vi "CheckCom2.vi"(11 "Data In":T2) -> (2 "States":T1, 3 "Data Out":T2)   [LabVIEW 2014]
uses:
  controls/Data.ctl
  controls/State.ctl
panel:
  # "日期"
  # "機種名稱"
  # "機種代號"
  # "商品條碼"
  # "台"
  # "OK"
  # "NG"
  # "台"
  # "總計"
  # "台"
  # "日期"
  # "機種名稱"
  # "機種代號"
  # "商品條碼"
  # "台"
  # "OK"
  # "NG"
  # "台"
  # "總計"
  # "台"
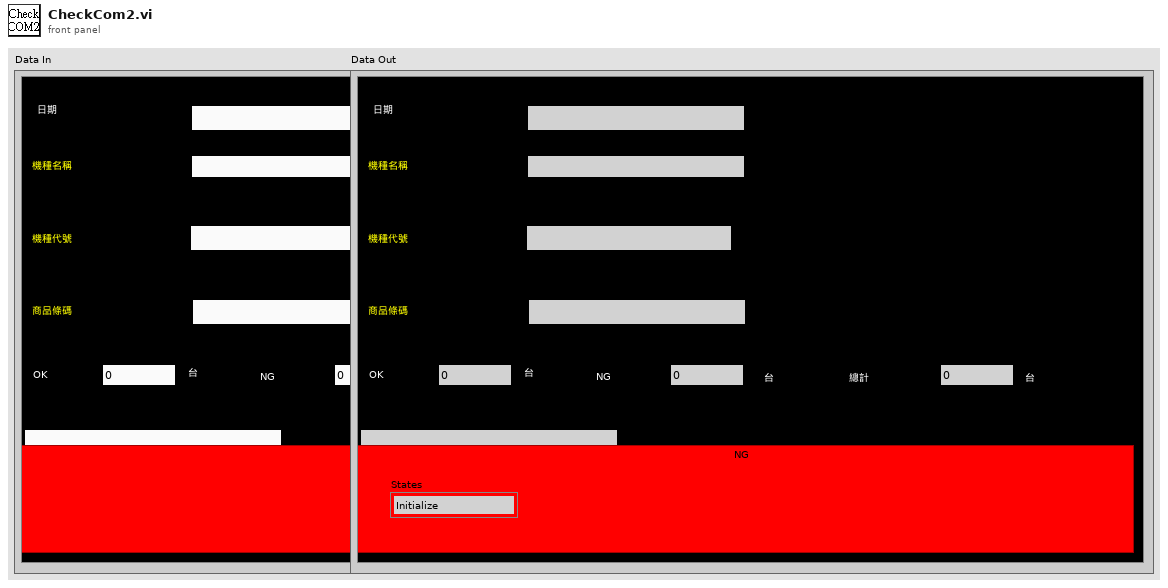
[diagram p1: front panel]
types:
  T1 = typedef "State.ctl" = enum16{"Initialize", "Wait for Scan", "State 1", "State 2", "NG", "OK", "OKNG", "Exit"}
  T2 = typedef "Data.ctl" = cluster{"Date":string, "BarCode1":string, "BarCode2":string, "BarCode3":string, "Message":string, "OK Count":u16, "NG Count":u16, "Total Count":u16, "ModelData":string[][], "OK&NG":bool, "COM1":refnum<visa-resource-name>, "COM2":refnum<visa-resource-name>, "IO":i32, "Time":u32, "TCP":refnum<k5>, "TCP 2":refnum<k5>}
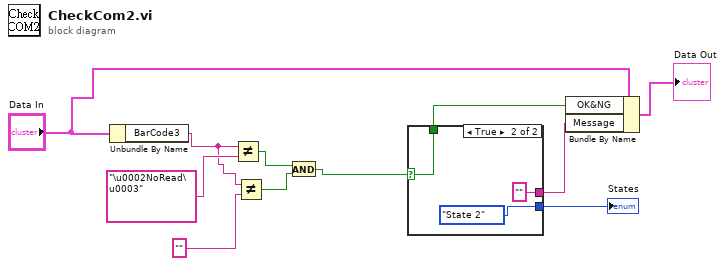
[diagram p0: block diagram]
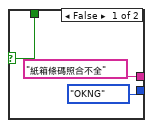
[diagram p2: hidden frame]
diagram:
  n1 = Unbundle By Name("Data In") -> ("BarCode3"=w5:string)
  n2 = Not Equal?(x=w5, y="\u0002NoRead\u0003") -> (x != y?=w3:bool)
  n3 = Not Equal?(x=w5, y="" ("f")) -> (x != y?=w2:bool)
  n4 = And(x=w3, y=w2) -> (x .and. y?=w1:bool)
  n5 = case shown="True" w1 {
    selector: w1 -> [w14 w17]
    tunnel: [w14 w17] -> w9
    tunnel: ["紙箱條碼照合不全" ""] -> w8
    tunnel: [State."OKNG" ("States") State."State 2" ("States")] -> w7
    frame False {
    }
    frame True {
    }
  }
  "States" <- w7
  n6 = Bundle By Name(cluster="Data In", "OK&NG"=w9, "Message"=w8) -> (→"Data Out":T2)
